vi "Make 3 chs Coincident.vi"(6 "interp. method":i32(ring) items=["nearest", "linear", "spline", "cubic Hermite", "Lagrange"], 9 "Time Cluster 3":T1, 10 "Time Cluster 2":T1, 11 "Time Cluster 1":T1) -> (1 "Coincident Time Cluster 3":T1, 2 "Coincident Time Cluster 2":T1, 3 "Coincident Time Cluster 1":T1)   [LabVIEW 2020]
uses:
  Controls/Time_Trace_Cluster.ctl
  <vilib>/Analysis/baseanly.llb/Mean (DBL).vi
  <vilib>/gmath/NI_Gmath.lvlib
  <vilib>/Analysis/NI_AALBase.lvlib
panel:
  in  "Number of Average Transit times":dbl=5.0 format="%#_13g"
  out "Time Window micro seconds":dbl
  out "Average TT":dbl format="%0.2f"
  out "Array":i32[](array[numeric])
  out "size(s)":i32
  in  "Show Plots":bool
  out "U1 and U2 Raw":cluster{"yi":dbl[], "yi":dbl[]}[](graph)
  out "U1 and U2 made coincident":cluster{"yi":dbl[], "yi":dbl[]}[](graph)
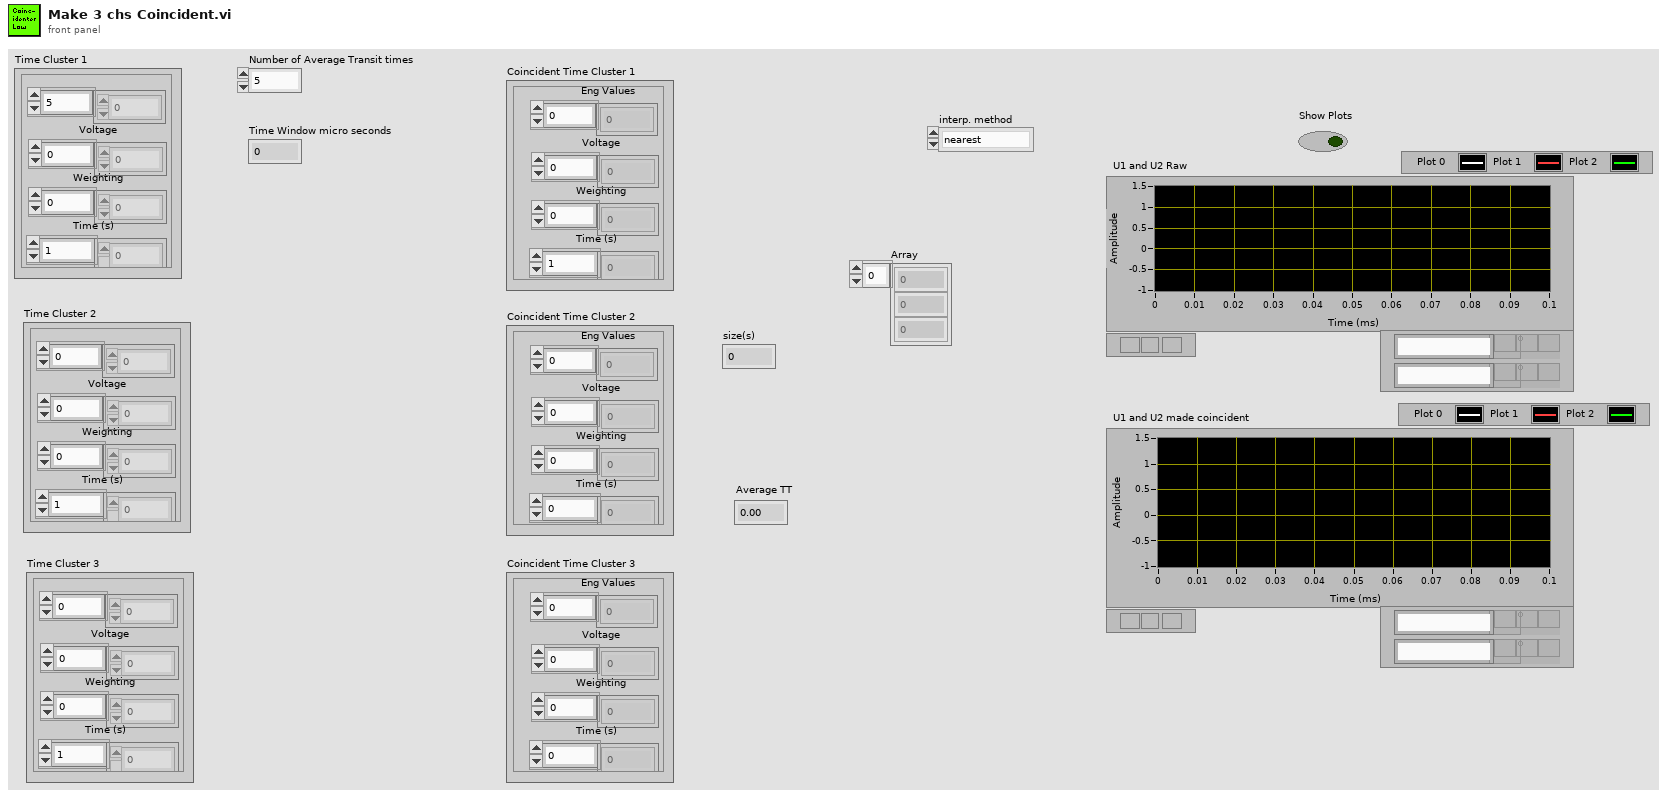
[diagram p1: front panel]
types:
  T1 = typedef "Time_Trace_Cluster.ctl" = cluster{"Weighting":dbl[], "Time (s)":dbl[], "Voltage":dbl[], "Eng Values":dbl[]}
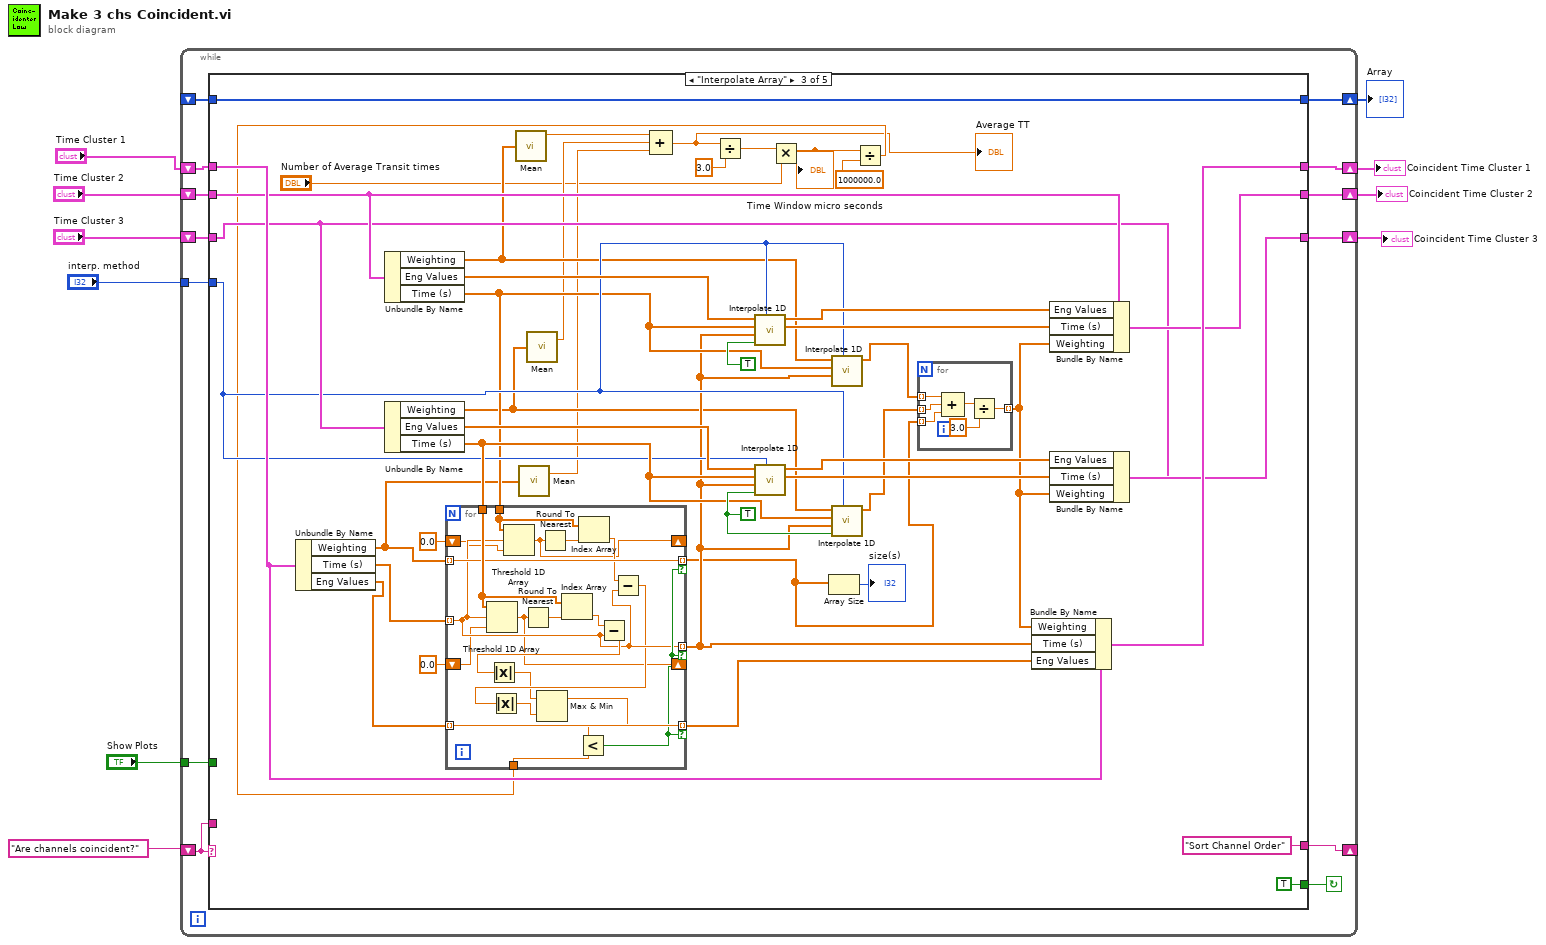
[diagram p0: block diagram]
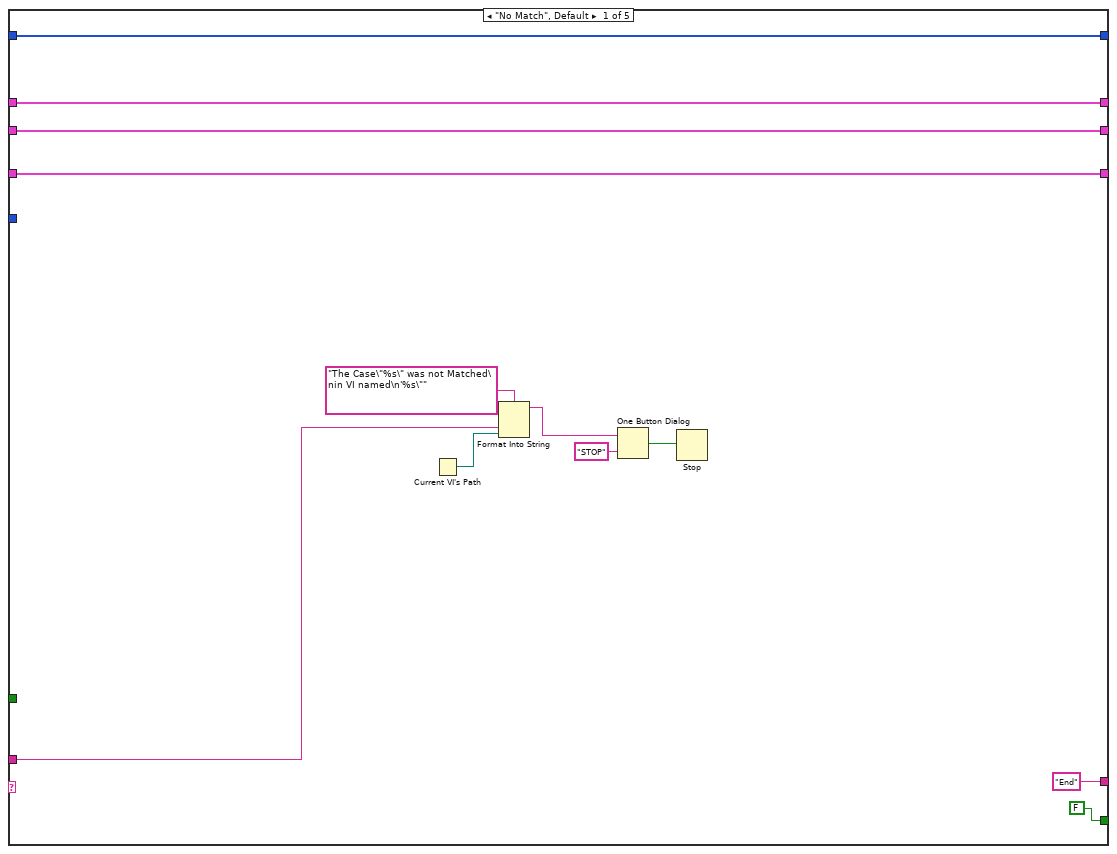
[diagram p2: hidden frame]
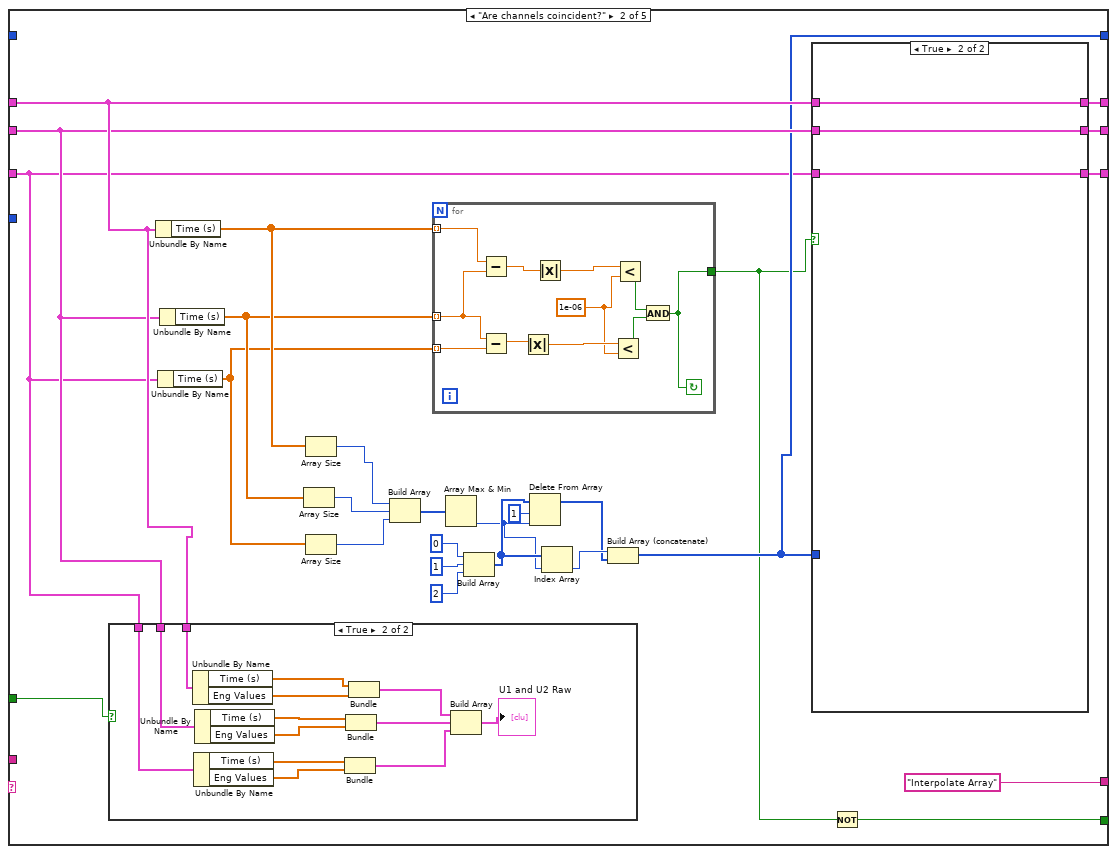
[diagram p3: hidden frame]
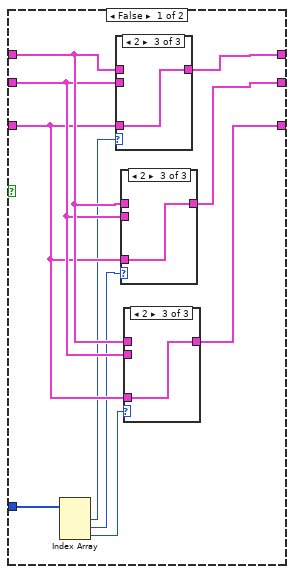
[diagram p4: hidden frame]
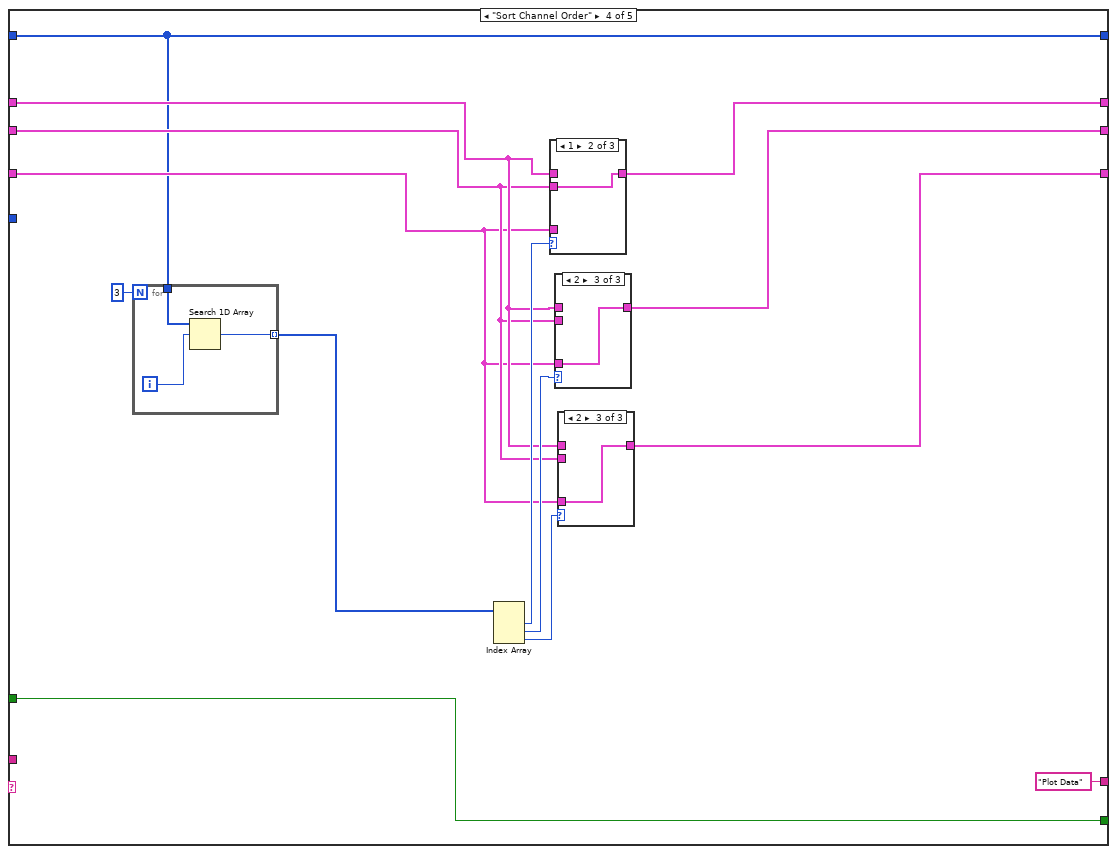
[diagram p12: hidden frame]
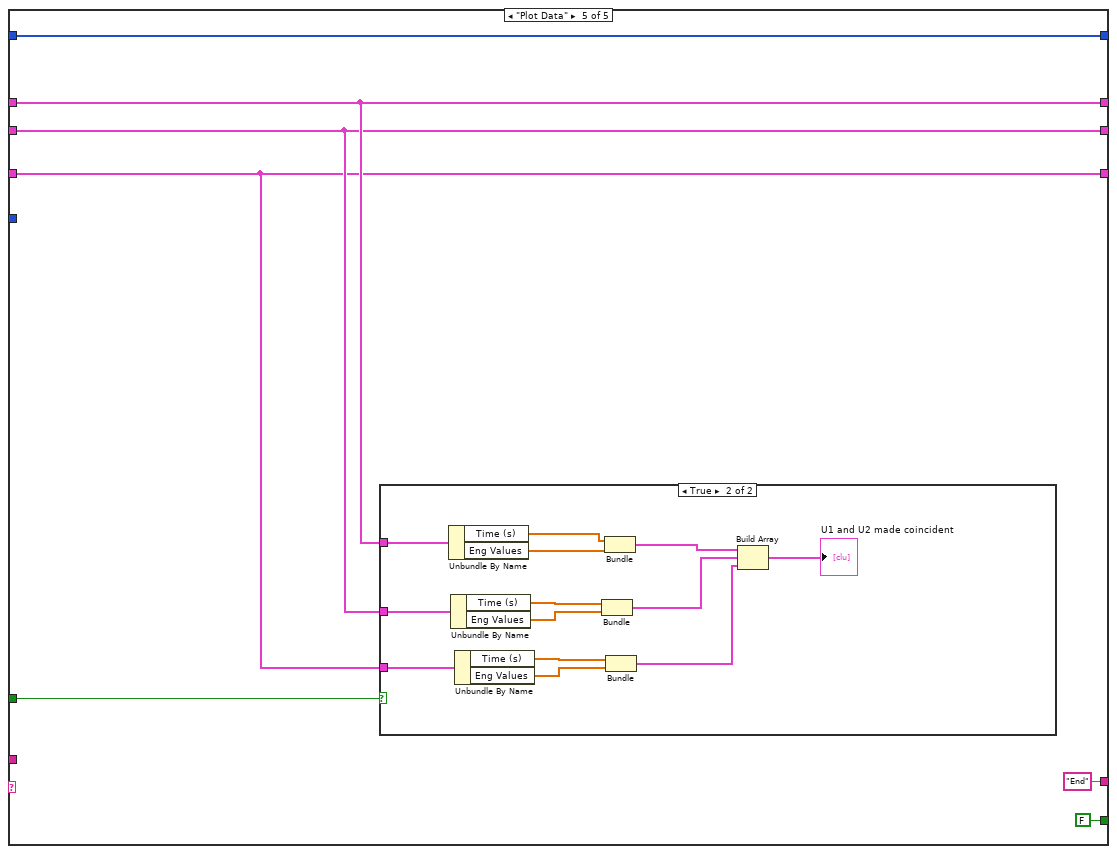
[diagram p19: hidden frame]
diagram:
  n1 = while {
    shift-right: [w18] -> w6
    shift-left: "Time Cluster 1" -> [w20]
    shift-right: [w17] -> w5
    shift-left: "Time Cluster 2" -> [w19]
    shift-right: [w21] -> _
    shift-left: "Are channels coincident?" -> [w23]
    tunnel: "Show Plots" -> [w16]
    shift-right: [w15] -> w1
    shift-left: _ -> [w14]
    tunnel: "interp. method" -> [w13]
    shift-right: [w11] -> w2
    shift-left: "Time Cluster 3" -> [w12]
    stop <- w22 continue-if-true
    n2 = case shown="\"Interpolate Array\"" w23 {
      tunnel: w23 -> [w30 _ _ _ _]
      tunnel: [FALSE w37 TRUE w180 FALSE] -> w22
      tunnel: ["End" "Interpolate Array" "Sort Channel Order" "Plot Data" ("t") "End" ("t")] -> w21
      tunnel: w20 -> [w27 w55 w142 w187 w207]
      tunnel: w19 -> [w26 w54 w132 w186 w206]
      tunnel: [w27 w57 w141 w184 w207] -> w18
      tunnel: [w26 w58 w134 w183 w206] -> w17
      tunnel: w16 -> [_ w56 _ w180 w208]
      tunnel: [w25 w39 w146 w178 w205] -> w15
      tunnel: w14 -> [w25 _ w146 w178 w205]
      tunnel: w13 -> [_ _ w130 _ _]
      tunnel: w12 -> [w24 w36 w131 w185 w204]
      tunnel: [w24 w40 w133 w182 w204] -> w11
      frame "No Match", Default {
        n3 = Current VI's Path() -> (path=w35:path)
        n4 = Format Into String(format string="The Case\"%s\" was not Matched\nin VI named\n'%s\"" ("Format String"), w30, w35) -> (resulting string=w32:string)  [unwired: 2 in, 1 out]
        n5 = One Button Dialog(message=w32, button name ("OK")="STOP") -> (true=w34:bool)
        n6 = Stop(stop? (T)=w34) -> ()
      }
      frame "Are channels coincident?" {
        n7 = case shown="True" w56 {
          tunnel: w55 -> [_ w89]
          tunnel: w54 -> [_ w88]
          tunnel: w36 -> [_ w86]
          frame False {
          }
          frame True {
            n8 = Unbundle By Name(w89) -> ("Time (s)"=w90:dbl[], "Eng Values"=w94:dbl[])
            n9 = Unbundle By Name(w86) -> ("Time (s)"=w85:dbl[], "Eng Values"=w87:dbl[])
            n10 = Unbundle By Name(w88) -> ("Time (s)"=w91:dbl[], "Eng Values"=w93:dbl[])
            n11 = Bundle("Time (s)"=w85, "Eng Values"=w87) -> (w84:cluster{"Time (s)":dbl[], "Eng Values":dbl[]})  [unwired: 1 in]
            n12 = Bundle("Time (s)"=w91, "Eng Values"=w93) -> (w92:cluster{"Time (s)":dbl[], "Eng Values":dbl[]})  [unwired: 1 in]
            n13 = Bundle("Time (s)"=w90, "Eng Values"=w94) -> (w95:cluster{"Time (s)":dbl[], "Eng Values":dbl[]})  [unwired: 1 in]
            n14 = Build Array(w95, w92, w84) -> (→"U1 and U2 Raw":cluster{"Time (s)":dbl[], "Eng Values":dbl[]}[])
          }
        }
        n15 = Unbundle By Name(w55) -> ("Time (s)"=w60:dbl[])
        n16 = Unbundle By Name(w36) -> ("Time (s)"=w53:dbl[])
        n17 = Unbundle By Name(w54) -> ("Time (s)"=w59:dbl[])
        n18 = Array Size(array=w59) -> (size(s)=w51:i32)
        n19 = Array Size(array=w60) -> (size(s)=w52:i32)
        n20 = Array Size(array=w53) -> (size(s)=w50:i32)
        n21 = Build Array(w52, w51, w50) -> (w49:i32[])
        n22 = for {
          tunnel: w60 -> [w105] mode=indexing
          tunnel: w59 -> [w104] mode=indexing
          tunnel: [w97] -> w38
          tunnel: w53 -> [w103] mode=indexing
          stop <- w97 continue-if-true
          w100 = 1e-06 ("y")
          n23 = Subtract(x=w105, y=w104) -> (x-y=w107:dbl)
          n24 = Subtract(x=w104, y=w103) -> (x-y=w102:dbl)
          n25 = Absolute Value(x=w102) -> (abs(x)=w101:dbl)
          n26 = Absolute Value(x=w107) -> (abs(x)=w106:dbl)
          n27 = Less?(x=w101, y=w100) -> (x < y?=w98:bool)
          n28 = Less?(x=w106, y=w100) -> (x < y?=w99:bool)
          n29 = And(x=w99, y=w98) -> (x .and. y?=w97:bool)
        }
        n30 = Array Max & Min(array=w49) -> (min index (indices)=w43:i32)  [unwired: 3 out]
        n31 = Build Array(0, 1, 2) -> (w44:i32[])
        n32 = Delete From Array(array=w44, length=1, index=w43) -> (array with subset deleted=w41:i32[])  [unwired: 1 out]
        n33 = Index Array(array=w44, index=w43) -> (element=w42:i32)
        n34 = Build Array (concatenate)(w42, w41) -> (w39:i32[])
        n35 = case shown="True" w38 {
          tunnel: [w71 w82] -> w58
          tunnel: [w70 w83] -> w57
          tunnel: w55 -> [w69 w83]
          tunnel: w54 -> [w68 w82]
          tunnel: [w65 w81] -> w40
          tunnel: w36 -> [w66 w81]
          tunnel: w39 -> [w67 _]
          frame False {
            n36 = Index Array(array=w67) -> (element #1=w64:i32, element #2=w63:i32, element #3=w62:i32)  [unwired: 3 in]
            n37 = case shown="2" w64 {
              tunnel: [w78 w79 w80] -> w70
              tunnel: w69 -> [w78 _ _]
              tunnel: w68 -> [_ w79 _]
              tunnel: w66 -> [_ _ w80]
              frame 0, Default {
              }
              frame 1 {
              }
              frame 2 {
              }
            }
            n38 = case shown="2" w63 {
              tunnel: [w75 w76 w77] -> w71
              tunnel: w69 -> [w75 _ _]
              tunnel: w68 -> [_ w76 _]
              tunnel: w66 -> [_ _ w77]
              frame 0, Default {
              }
              frame 1 {
              }
              frame 2 {
              }
            }
            n39 = case shown="2" w62 {
              tunnel: [w72 w73 w74] -> w65
              tunnel: w69 -> [w72 _ _]
              tunnel: w68 -> [_ w73 _]
              tunnel: w66 -> [_ _ w74]
              frame 0, Default {
              }
              frame 1 {
              }
              frame 2 {
              }
            }
          }
          frame True {
          }
        }
        n40 = Not(x=w38) -> (.not. x?=w37:bool)
      }
      frame "Interpolate Array" {
        w140 = TRUE ("X is monotonic")
        n41 = Unbundle By Name(w142) -> ("Weighting"=w118:dbl[], "Time (s)"=w145:dbl[], "Eng Values"=w143:dbl[])
        n42 = Unbundle By Name(w132) -> ("Weighting"=w120:dbl[], "Eng Values"=w135:dbl[], "Time (s)"=w129:dbl[])
        n43 = Unbundle By Name(w131) -> ("Weighting"=w119:dbl[], "Eng Values"=w151:dbl[], "Time (s)"=w139:dbl[])
        n44 = call-poly <vilib>:"Mean.vi"("X"=w120) -> ("mean"=w116:dbl)  [unwired: 1 out]
        n45 = call-poly <vilib>:"Mean.vi"("X"=w118) -> ("mean"=w115:dbl)  [unwired: 1 out]
        n46 = call-poly <vilib>:"Mean.vi"("X"=w119) -> ("mean"=w114:dbl)  [unwired: 1 out]
        n47 = Compound Arithmetic op=ADD(w116, w114, w115) -> (w108:dbl)
        "Average TT" <- w108
        n48 = Divide(x=w108, y=3.0) -> (x/y=w113:dbl)
        n49 = Multiply(x=w113, y="Number of Average Transit times") -> (x*y=w111:dbl)
        "Time Window micro seconds" <- w111
        n50 = Divide(x=w111, y=1000000.0) -> (x/y=w109:dbl)
        n51 = for {
          tunnel: w145 -> [w166] mode=indexing
          tunnel: w139 -> [w176]
          tunnel: [w166] -> w128 mode=indexing if=w172
          tunnel: [w174] -> w144 mode=indexing if=w172
          tunnel: w143 -> [w174] mode=indexing
          tunnel: [w173] -> w124 mode=indexing if=w172
          tunnel: w118 -> [w173] mode=indexing
          tunnel: w109 -> [w171]
          tunnel: w129 -> [w169]
          shift-right: [w160] -> _
          shift-left: 0.0 -> [w161]
          shift-right: [w158] -> _
          shift-left: 0.0 -> [w159]
          n52 = Threshold 1D Array(1:w159, 2:w166, 3:w176) -> (0:w158:dbl)
          n53 = Threshold 1D Array(1:w161, 2:w166, 3:w169) -> (0:w160:dbl)
          n54 = Round To Nearest(number=w158) -> (nearest integer value=w177:dbl)
          n55 = Round To Nearest(number=w160) -> (nearest integer value=w170:dbl)
          n56 = Index Array(array=w176, index=w177) -> (element=w175:dbl)
          n57 = Index Array(array=w169, index=w170) -> (element=w167:dbl)
          n58 = Subtract(x=w175, y=w166) -> (x-y=w168:dbl)
          n59 = Absolute Value(x=w168) -> (abs(x)=w164:dbl)
          n60 = Subtract(x=w167, y=w166) -> (x-y=w165:dbl)
          n61 = Absolute Value(x=w165) -> (abs(x)=w163:dbl)
          n62 = Max & Min(x=w164, y=w163) -> (max(x,y)=w162:dbl)  [unwired: 1 out]
          n63 = Less?(x=w162, y=w171) -> (x < y?=w172:bool)
        }
        n64 = call <vilib>:"Interpolate 1D.vi"("method"=w130, "X is monotonic"=TRUE, "xi"=w128, "X"=w129, "Y"=w135) -> ("xi used"=w137:dbl[], "yi"=w136:dbl[])  [unwired: 1 in, 4 out]
        n65 = call <vilib>:"Interpolate 1D.vi"("method"=w130, "X is monotonic"=w140, "xi"=w128, "X"=w139, "Y"=w151) -> ("xi used"=w149:dbl[], "yi"=w150:dbl[])  [unwired: 1 in, 4 out]
        n66 = Array Size(array=w124) -> (size(s)=→"size(s)":i32)
        n67 = call <vilib>:"Interpolate 1D.vi"("method"=w130, "xi"=w128, "X"=w129, "Y"=w120) -> ("yi"=w126:dbl[])  [unwired: 2 in, 5 out]
        n68 = call <vilib>:"Interpolate 1D.vi"("method"=w130, "X is monotonic"=w140, "xi"=w128, "X"=w139, "Y"=w119) -> ("yi"=w125:dbl[])  [unwired: 1 in, 5 out]
        n69 = for {
          tunnel: w126 -> [w157] mode=indexing
          tunnel: w125 -> [w156] mode=indexing
          tunnel: w124 -> [w155] mode=indexing
          tunnel: [w152] -> w121 mode=indexing
          n70 = Compound Arithmetic op=ADD(w157, w156, w155) -> (w154:dbl)
          n71 = Divide(x=w154, y=3.0) -> (x/y=w152:dbl)
        }
        n72 = Bundle By Name(cluster=w142, "Weighting"=w121, "Time (s)"=w128, "Eng Values"=w144) -> (w141:T1)
        n73 = Bundle By Name(cluster=w132, "Eng Values"=w136, "Time (s)"=w137, "Weighting"=w121) -> (w134:T1)
        n74 = Bundle By Name(cluster=w131, "Eng Values"=w150, "Time (s)"=w149, "Weighting"=w121) -> (w133:T1)
      }
      frame "Sort Channel Order" {
        n75 = for {
          N: 3 -> [_]
          tunnel: w178 -> [w202]
          tunnel: [w201] -> w188 mode=indexing
          i -> [w203]
          n76 = Search 1D Array(1D array=w202, element=w203) -> (index of element=w201:i32)  [unwired: 1 in]
        }
        n77 = Index Array(array=w188) -> (element #1=w191:i32, element #2=w190:i32, element #3=w189:i32)  [unwired: 3 in]
        n78 = case shown="1" w191 {
          tunnel: [w198 w199 w200] -> w184
          tunnel: w187 -> [w198 _ _]
          tunnel: w186 -> [_ w199 _]
          tunnel: w185 -> [_ _ w200]
          frame 0, Default {
          }
          frame 1 {
          }
          frame 2 {
          }
        }
        n79 = case shown="2" w190 {
          tunnel: [w195 w196 w197] -> w183
          tunnel: w187 -> [w195 _ _]
          tunnel: w186 -> [_ w196 _]
          tunnel: w185 -> [_ _ w197]
          frame 0, Default {
          }
          frame 1 {
          }
          frame 2 {
          }
        }
        n80 = case shown="2" w189 {
          tunnel: [w192 w193 w194] -> w182
          tunnel: w187 -> [w192 _ _]
          tunnel: w186 -> [_ w193 _]
          tunnel: w185 -> [_ _ w194]
          frame 0, Default {
          }
          frame 1 {
          }
          frame 2 {
          }
        }
      }
      frame "Plot Data" {
        n81 = case shown="True" w208 {
          tunnel: w207 -> [_ w223]
          tunnel: w206 -> [_ w222]
          tunnel: w204 -> [_ w212]
          frame False {
          }
          frame True {
            n82 = Unbundle By Name(w223) -> ("Time (s)"=w216:dbl[], "Eng Values"=w220:dbl[])
            n83 = Unbundle By Name(w222) -> ("Time (s)"=w217:dbl[], "Eng Values"=w219:dbl[])
            n84 = Unbundle By Name(w212) -> ("Time (s)"=w214:dbl[], "Eng Values"=w213:dbl[])
            n85 = Bundle("Time (s)"=w217, "Eng Values"=w219) -> (w218:cluster{"Time (s)":dbl[], "Eng Values":dbl[]})  [unwired: 1 in]
            n86 = Bundle("Time (s)"=w216, "Eng Values"=w220) -> (w221:cluster{"Time (s)":dbl[], "Eng Values":dbl[]})  [unwired: 1 in]
            n87 = Bundle("Time (s)"=w214, "Eng Values"=w213) -> (w211:cluster{"Time (s)":dbl[], "Eng Values":dbl[]})  [unwired: 1 in]
            n88 = Build Array(w221, w218, w211) -> (→"U1 and U2 made coincident":cluster{"Time (s)":dbl[], "Eng Values":dbl[]}[])
          }
        }
      }
    }
  }
  "Coincident Time Cluster 1" <- w6
  "Coincident Time Cluster 2" <- w5
  "Coincident Time Cluster 3" <- w2
  "Array" <- w1
